vi "读取参数表格文件样例.vi"(9 "下载路径":path=path "D:/项目/MPZ2006_solid source/数据模版/参数表格文件样例.xlsx") -> (2 "data":string[][](array[string]))   [LabVIEW 2015]
uses:
  <vilib>/addons/_office/excel.llb/Excel Get Data ([str]).vi
  <vilib>/Utility/NIReport.llb/NI_report.lvclass
  <vilib>/addons/_office/NI_ReportGenerationToolkit.lvlib
  <vilib>/Utility/NIReport.llb/Excel/NI_Excel.lvclass
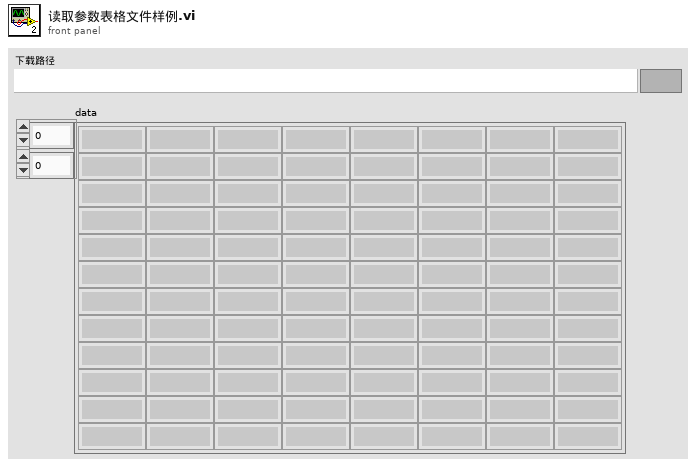
[diagram p1: front panel]
types:
  T1 = enum16{"Standard Report", "HTML", "Word", "Excel"}
  T2 = enum16{"maximized", "minimized", "normal", "no change"}
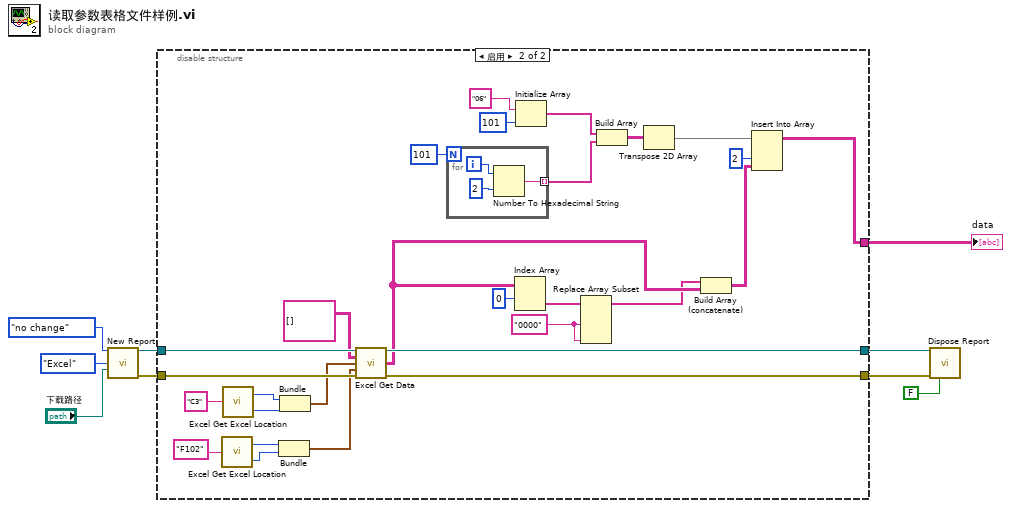
[diagram p0: block diagram]
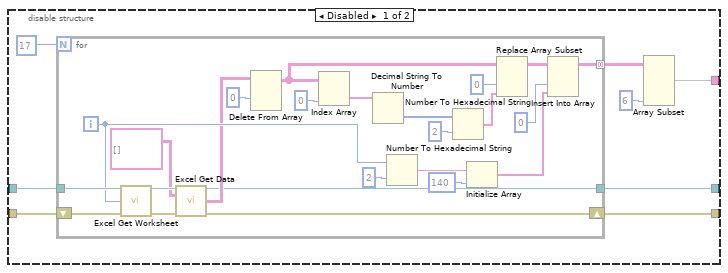
[diagram p2: hidden frame]
diagram:
  n1 = call <vilib>:"New Report.vi"("window state (normal)"=T2."no change", "report type"=T1."Excel", "template (empty)"="下载路径") -> ("report out"=w5:refnum<class "NI_report.lvclass">, "error out"=w6:errorcluster)  [unwired: 11 in]
  n2 = disable-structure shown="启用" {
    disable-tunnel: w6 -> [w17 w68]
    disable-tunnel: w5 -> [w16 w69]
    disable-tunnel: [w14 w58] -> w4
    disable-tunnel: [w13 w57] -> w3
    disable-tunnel: [w10 w43] -> w1
    frame Disabled {
      n3 = for {
        N: 17 -> [_]
        tunnel: w16 -> [w41]
        tunnel: [w28] -> w12 mode=concatenating
        tunnel: [w27] -> w14
        shift-right: [w26] -> w13
        shift-left: w17 -> [w40]
        i -> [w36]
        n4 = call <vilib>:"Excel Get Worksheet.vi"("report in"=w41, "worksheet index (0)"=w36, "error in (no error)"=w40) -> ("report out"=w38:refnum<class "NI_report.lvclass">, "error out"=w39:errorcluster)  [unwired: 11 in]
        n5 = call-poly <vilib>:"Excel Get Data.vi"("report in"=w38, "data type"=string[][] [], "error in (no error)"=w39) -> ("report out"=w27:refnum<class "NI_report.lvclass">, "data"=w33:string[][], "error out"=w26:errorcluster)  [unwired: 10 in]
        n6 = Delete From Array(array=w33, index (row)=0 ("索引 (行)")) -> (array with subset deleted=w21:string[][])  [unwired: 2 in, 1 out]
        n7 = Index Array(array=w21, index (col)=0 ("禁用的索引 (列)")) -> (element=w24:string[])  [unwired: 1 in]
        n8 = Decimal String To Number(string=w24) -> (number=w23:i32[])  [unwired: 2 in, 1 out]
        n9 = Number To Hexadecimal String(1:i16 2 ("宽度(-)"), 2:w36) -> (0:w32:string)
        n10 = Number To Hexadecimal String(1:i16 2 ("宽度(-)"), 2:w23) -> (0:w20:string[])
        n11 = Initialize Array(w32, 140 ("维数大小")) -> (w30:string[])
        n12 = Replace Array Subset(array=w21, new element=w20, index (col)=0 ("禁用的索引 (列)")) -> (w18:string[][])  [unwired: 1 in]
        n13 = Insert Into Array(array=w18, index (col)=0 ("禁用的索引 (列)"), new element=w30) -> (w28:string[][])  [unwired: 1 in]
      }
      n14 = Array Subset(array=w12, length (col)=6 ("长度")) -> (w10:string[][])  [unwired: 3 in]
    }
    frame Enabled {
      w54 = "0000" ("新元素/子数组")
      n15 = call <vilib>:"Excel Get Excel Location.vi"("cell's name"="F102") -> ("row"=w60:i32, "column"=w61:i32)
      n16 = call <vilib>:"Excel Get Excel Location.vi"("cell's name"="C3") -> ("row"=w64:i32, "column"=w63:i32)
      n17 = Bundle("row"=w60, "column"=w61) -> (w59:cluster{"row":i32, "column":i32})  [unwired: 1 in]
      n18 = Bundle("row"=w64, "column"=w63) -> (w62:cluster{"row":i32, "column":i32})  [unwired: 1 in]
      n19 = call-poly <vilib>:"Excel Get Data.vi"("report in"=w69, "data type"=string[][] [], "start (-1, -1)"=w62, "end (-1, -1)"=w59, "error in (no error)"=w68) -> ("report out"=w58:refnum<class "NI_report.lvclass">, "data"=w53:string[][], "error out"=w57:errorcluster)  [unwired: 8 in]
      n20 = for {
        N: 101 -> [_]
        tunnel: [w70] -> w47 mode=indexing
        i -> [w71]
        n21 = Number To Hexadecimal String(1:i16 2 ("宽度(-)"), 2:w71) -> (0:w70:string)
      }
      n22 = Index Array(array=w53, index (row)=0 ("索引 (行)")) -> (element=w55:string[])  [unwired: 1 in]
      n23 = Initialize Array("06" ("新元素/子数组"), 101 ("维数大小")) -> (w48:string[])
      n24 = Replace Array Subset(array=w55, new element #1=w54, new element #2=w54) -> (w52:string[])  [unwired: 2 in]
      n25 = Build Array(w48, w47) -> (w46:string[][])
      n26 = Transpose 2D Array(2D array=w46) -> (transposed array=w45:string[][])
      n27 = Build Array (concatenate)(w52, w53) -> (w44:string[][])
      n28 = Insert Into Array(array=w45, index (col)=2 ("禁用的索引 (列)"), new element=w44) -> (w43:string[][])  [unwired: 1 in]
    }
  }
  "data" <- w1
  n29 = call-dynamic "Dispose Report.vi"("report in"=w4, "error in (no error)"=w3, "close report? (T)"=FALSE) -> ()  [unwired: 12 in, 1 out]
